vi "DefenseKick.vi"(0 "object in":refnum<class "DefendAreaTactic.lvclass">, 2 "Robot":refnum<class "Robot.lvclass">, 4 "Game":refnum<class "Game.lvclass">, 5 "error in (no error)":errorcluster) -> (14 "object out":refnum<class "DefendAreaTactic.lvclass">, 16 "Robot out":refnum<class "Robot.lvclass">, 19 "error out":errorcluster)   [LabVIEW 2024, in "DefendAreaTactic.lvclass"]
doc: "Defenders kick ball away when it is close."
uses:
  DefendAreaTactic.lvclass
  Game_class/Game.lvclass
  Robot_class/Robot.lvclass
  Game_class/Game.lvclass/Game.ctl
  Parameters_class/Parameters.lvclass/Parameters.ctl
  Robot_class/Robot.lvclass/Robot.ctl
  Game_class/Read Utilities.lvclass.vi
  Game_class/Read FieldRef.vi
  Game_class/Read BallRef.vi
  Robot_class/Read id.vi
  Robot_class/Write kick_x.vi
  Robot_class/Write kick_z.vi
  Robot_class/Read orientation.vi
  Game_class/Read NewParameters.vi
  Game_class/Read Parameters.lvclass.vi
  Parameters_class/Read minDistanceToPass.vi
  Parameters_class/Read Enviroment.vi
  Parameters_class/Read MinDistToKick.vi
  Parameters_class/Read ChipKick activated.vi
  Parameters_class/Read ChipKick Force 1.vi
  Parameters_class/Read KickForce.vi
  Parameters_class/Read PassForceMult.vi
  Parameters_class/Parameters.lvclass
  Ball_class/Ball.lvclass
  Utilities_class/Utilities.lvclass
  Field_class/Field.lvclass
  KickToSkill_class/KickToSkill.lvclass
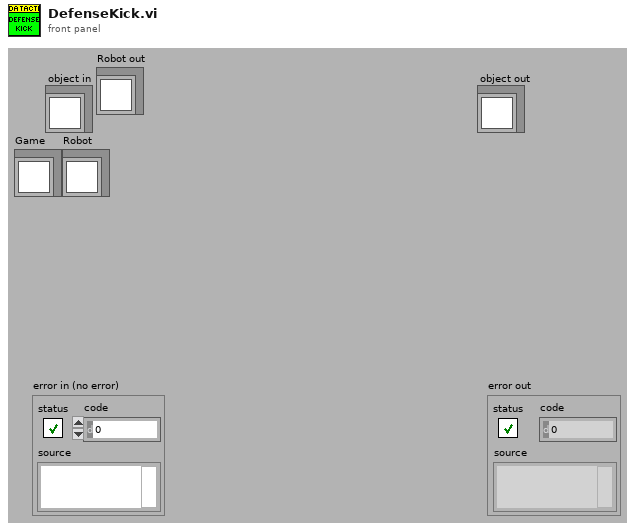
[diagram p1: front panel]
types:
  T1 = typedef "NewParameters.ctl" = cluster{"PenaltyDistance":dbl, "DistanceAttackerToBackBall":dbl, "Division":enum16{"Div B", "Div A"}, "DistanceToAvoidyEnemyRobot":dbl, "BallPlacementDistance":dbl, "DisatanceBehindBallToStealBall":dbl, "MaxDistanceToPositionKickoff":dbl, "BlockEnemyTarget":bool, "MaxStopVAng":dbl, "DistanceMarkerToEnemy":dbl, "IgnoreDribblerContact":bool, "DistanceToBeginEnemyPosession":dbl, "GoToBallWhenEnemyNotMoving":bool, "EnemyDistanceToReduceVelocity":dbl, "TurnOnEnemyDistanceToReduceVelocity":bool, "EnemyDistanceToShootOutBall":dbl, "DefenseKickBall":bool, "MoreKickToGoal? (0-0.3)":dbl, "ChipKickInEnemyField":bool, "ShootOutRobotId":dbl, "FieldLenghtDenominatorInShootOut":dbl, "AdjustPositionInBallPlacement":bool, "PowerGodPass":dbl, "VelocityAbortEnemyPos":dbl, "MaxDistToBeginPass":dbl, "MinDistToBeginPass":dbl, "VelocityInDirects":dbl, "BadDribblerIDs":i32[], "NewKickToDistanceAroundBall":dbl, "PowerAvoidColisionMarker":dbl, "DistanceToAvoidColisionMarker":dbl, "AvoidBallKick":dbl, "DistanceTryKick":dbl, "SuicideKickDIstance":dbl, "AdjustFirstKickDistance":dbl, "AvoidAimLessKick":dbl, "DistanceToAvoidyEnemyShootRobot ":dbl, "NumberOfMarkers":dbl, "PotField":bool, "PIDLateral":bool, "MinDistanceFirstKickX":dbl, "MinDistanceFirstKickY":dbl, "FractionOfDistToTouchGround\nAfterChipKick":dbl, "FractionOfKickxWhen\nComposedWithKickz":dbl, "Style":T2, "MoveInTurnState":bool, "DistFromEnemyToConsider\nMoveInTurnState":dbl, "CascadePID":bool, "TurnAroundParameters":cluster{"Radius":dbl, "Multiplier":dbl, "ChordAngle":dbl}, "SafeDriveVel":dbl, "DistanceToGoToBackBall":dbl, "minDistanceToNotFinish\nEnemyPossession":dbl, "OneTouchShot":cluster{"angleFactor":dbl, "maxAngle":dbl, "Attack":bool, "Defense":bool}, "OpenAngleToGoal":cluster{"minAngle":dbl, "maxAngle":dbl, "minEvaluation":dbl}, "ShotInterception":cluster{"shotSpeed":dbl, "minEnemySpeed":dbl, "maxEnemySpeed":dbl, "minEvaluation":dbl}, "AllyTeamArray":T3[], "maxDefendersNumber":i32, "Zone":cluster{"GuardPositionArray":dbl[][], "ZoneMidField":dbl[], "CenterForwardWidth":dbl}, "MinEvaluationToShoot":dbl, "PassInterception":cluster{"maxPassSpeed":dbl, "minPassSpeed":dbl, "minEnemySpeed":dbl, "chipPassDistance":dbl, "chipPassEvaluation":dbl, "minEvaluation":dbl, "maxEnemySpeed":dbl}, "PassDistance":cluster{"maxDistance":dbl, "minDistance":dbl}, "receiverSpeed":dbl, "maxBallSpeed":dbl, "slackTime":dbl, "Turning radius":dbl, "Turning v_ang":dbl, "AlignError":cluster{"Distance":dbl, "Orientation":dbl, "V_norm(m/s)":dbl, "V_ang (rad/s)":dbl}, "RobotRadius":dbl, "KickerDistance":dbl, "keeper angle  to cover goalpost":dbl, "a_slide":dbl, "a_roll":dbl, "k_switch":dbl, "Penalty":u16}
  T2 = typedef "Style.ctl" = enum16{"Insanity", "Offensive", "Defensive"}
  T3 = typedef "AllyTeam.ctl" = enum16{"Keeper", "Defender", "Attacker"}
  T4 = typedef "Enviroment.ctl" = enum16{"erForceSimulator", "grSim", "realGame"}
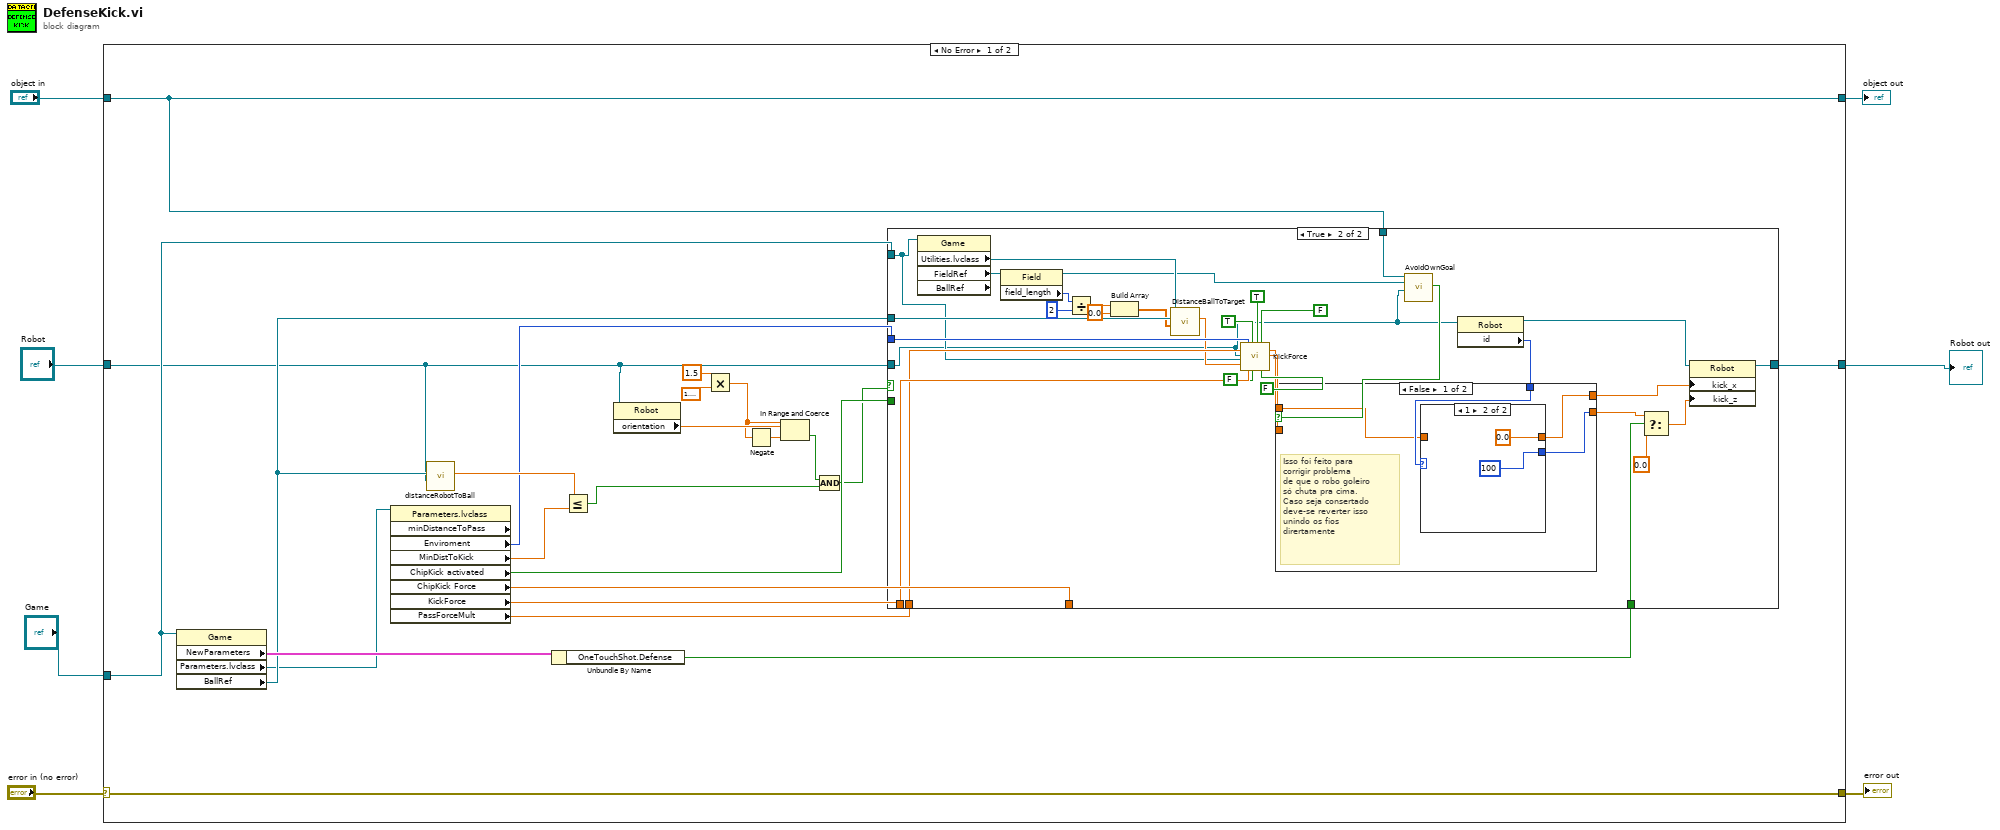
[diagram p0: block diagram]
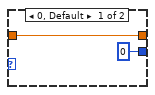
[diagram p3: hidden frame]
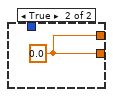
[diagram p4: hidden frame]
diagram:
  n1 = case shown="No Error" "error in (no error)" {
    selector: "error in (no error)" -> [w31 w76]
    tunnel: [w31 w76] -> w6
    tunnel: [w14 w75] -> w4
    tunnel: "object in" -> [w14 w75]
    tunnel: "Game" -> [w13 _]
    tunnel: "Robot" -> [w10 w74]
    tunnel: [w9 w74] -> w1
    frame No Error {
      n2 = property class="Game"(reference=w13) -> ("NewParameters"=w21:T1, "Parameters.lvclass"=w11:refnum<class "Parameters.lvclass">, "BallRef"=w12:refnum<class "Ball.lvclass">)  [unwired: 1 in, 2 out]
      n3 = property class="Parameters.lvclass" props=["minDistanceToPass", "Enviroment", "MinDistToKick", "ChipKick activated", "ChipKick Force", "KickForce", "PassForceMult"](reference=w11) -> ("Enviroment"=w26:T4, "MinDistToKick"=w29:dbl, "ChipKick activated"=w28:bool, "ChipKick Force"=w27:dbl, "KickForce"=w25:dbl, "PassForceMult"=w24:dbl)  [unwired: 1 in, 3 out]
      n4 = call "distanceRobotToBall.vi"("Robot"=w10, "Ball"=w12) -> ("Distance Robot To Ball"=w30:dbl)  [unwired: 7 in, 2 out]
      n5 = Unbundle By Name(w21) -> ("OneTouchShot.Defense"=w8:bool)
      n6 = Less Or Equal?(x=w30, y=w29) -> (x <= y?=w22:bool)
      n7 = property class="Robot"(reference=w10) -> ("orientation"=w20:dbl)  [unwired: 1 in, 2 out]
      n8 = Multiply(x=1.5, y=1.5707963267948966) -> (x*y=w15:dbl)
      n9 = Negate(x=w15) -> (-x=w19:dbl)
      n10 = In Range and Coerce(upper limit=w15, x=w20, lower limit=w19) -> (In Range?=w18:bool)  [unwired: 1 out]
      n11 = Compound Arithmetic op=AND(w18, w22) -> (w23:bool)
      n12 = case shown="True" w23 {
        tunnel: w10 -> [w32 w35]
        tunnel: w28 -> [_ _]
        tunnel: w27 -> [_ _]
        tunnel: w26 -> [_ w63]
        tunnel: w25 -> [_ w61]
        tunnel: w24 -> [_ w60]
        tunnel: w12 -> [_ w59]
        tunnel: w13 -> [_ w49]
        tunnel: w14 -> [_ w40]
        tunnel: [w32 w64] -> w9
        tunnel: w8 -> [_ w39]
        frame False {
        }
        frame True {
          n13 = property class="Game" props=["Utilities.lvclass", "FieldRef", "BallRef"](reference=w49) -> ("Utilities.lvclass"=w51:refnum<class "Utilities.lvclass">, "FieldRef"=w57:refnum<class "Field.lvclass">)  [unwired: 1 in, 3 out]
          n14 = property class="Field"(reference=w57) -> (reference out=w42:refnum<class "Field.lvclass">, "field_length"=w56:i32)  [unwired: 1 in, 1 out]
          n15 = Divide(x=w56, y=2) -> (x/y=w54:dbl)
          n16 = Build Array(w54, 0.0 ("element")) -> (w53:dbl[])
          n17 = call "DistanceBallToTarget.vi"("Target"=w53, "Ball"=w59, "Utilities in"=w51) -> ("Distance Ball To Target"=w58:dbl)  [unwired: 6 in, 2 out]
          n18 = call "KickForce.vi"("force++"=w60, "Robot"=w35, "Game"=w49, "Distance to target"=w58, "Enviroment"=w63, "kickForce"=w61, "chipKick ?"=TRUE, "weakKick?"=FALSE, "shootState?"=TRUE, "use criteria?"=FALSE, "pass?"=FALSE) -> ("kick_x Force out"=w43:dbl, "kick_z Force out"=w44:dbl)  [unwired: 5 in, 2 out]
          n19 = call "AvoidOwnGoal.vi"("DefendAreaTactic in"=w40, "Field"=w42, "Robot"=w35) -> ("Is shooting to our goal?"=w41:bool)  [unwired: 14 in, 2 out]
          n20 = property class="Robot"(reference=w35) -> (reference out=w34:refnum<class "Robot.lvclass">, "id"=w33:i32)  [unwired: 1 in, 1 out]
          n21 = case shown="False" w41 {
            tunnel: [w66 w73] -> w45
            tunnel: [w67 w73] -> w38
            tunnel: w44 -> [_ _]
            tunnel: w43 -> [w65 _]
            tunnel: w33 -> [w68 _]
            frame False {
              # "Isso foi feito para\ncorrigir problema\nde que o robo goleiro\nsó chuta pra cima.\nCaso seja consertado\ndeve-se reverter isso\nunindo os fios dirertamente"
              n22 = case shown="1" w68 {
                tunnel: [0 100] -> w67
                tunnel: [w69 0.0] -> w66
                tunnel: w65 -> [w69 _]
                frame 0, Default {
                }
                frame 1 {
                }
              }
            }
            frame True {
              w73 = 0.0
            }
          }
          n23 = Select(t=w38, s=w39, f=0.0) -> (s? t:f=w37:dbl)
          n24 = property class="Robot"(reference=w34, "kick_x"=w45, "kick_z"=w37) -> (reference out=w64:refnum<class "Robot.lvclass">)  [unwired: 1 in, 1 out]
        }
      }
    }
    frame Error {
    }
  }
  "error out" <- w6
  "object out" <- w4
  "Robot out" <- w1
